vi "StringToTimeStamp.vi"(8 "error in (no error)":errorcluster, 10 "TimeStamp":string) -> (0 "error out":errorcluster, 2 "Time Stamp":timestamp)   [LabVIEW 2015, in "Request.lvclass"]
uses:
  Request.lvclass
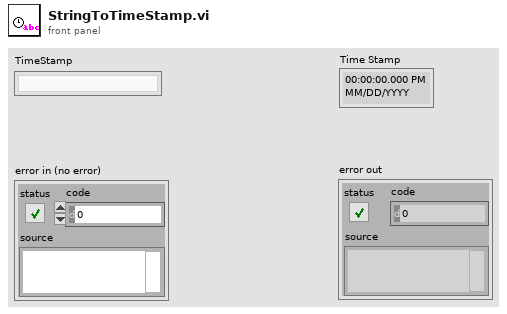
[diagram p1: front panel]
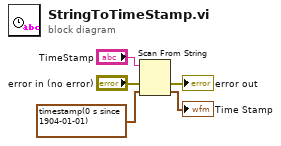
[diagram p0: block diagram]
diagram:
  n1 = Scan From String(input string="TimeStamp", error in="error in (no error)", default 1=timestamp(0 s since 1904-01-01) ("Time Stamp")) -> (error out=→"error out":errorcluster, output 1=→"Time Stamp":timestamp)  [unwired: 2 in, 2 out]
